vi "PID Servo Position.vi"() -> ()   [LabVIEW 2012]
doc: "<B>PID Servo Position</B> implements PID control of the Camera Servo Motor."
uses:
  <vilib>/Rock Robotics/SystemInterfaces/DIO/FPGA_DIOPWMChannel.ctl
  <vilib>/Rock Robotics/SystemInterfaces/Typedef/FPGA_TypedefDigitalModule.ctl
  <vilib>/addons/control/pid/pid.llb/PID (DBL).vi
  <vilib>/addons/control/pid/NI_PID_pid.lvlib
panel:
  in  "PID gains":T1={"proportional gain (Kc)"=1.0, "integral time (Ti, min)"=0.01, "derivative time (Td, min)"=0.0} {"derivative time (Td, min)" format="%.3f"; "integral time (Ti, min)" format="%.3f"; "proportional gain (Kc)" format="%.3f"}
  in  "Desired Angle":dbl format="%.2f"
  in  "PWM Channel":T2=enum."PWM 6"
  out "Current Angle":u16(knob) scale=0.0..170.0
  in  "stop":bool
  # "1. Select the PWM channel for the servo.\n2. Press the run button\n3. Adjust the PID Gains\n4. Set your Desired Angle\n5. The Current Angle is displayed in the dial\n6. Press STOP to end the program"
  # "Wiring Diagram for Digital Sidecar connected to an NI 9403"
  # "power jumper required for servo"
  # "The black wire should go into ground (-).\nThe red wire should go to power (PWR)\nThe white or yellow wire should go to signal (SIG)"
  # "PWR"
  # "SIG"
  # "(-)"
  # "+V"
  # "10"
  # "9"
  # "8"
  # "7"
  # "6"
  # "5"
  # "4"
  # "3"
  # "2"
  # "1"
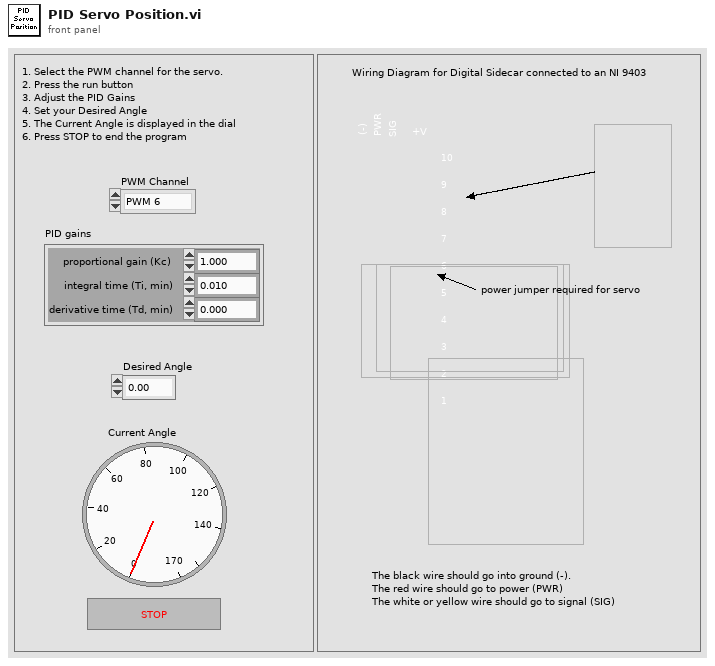
[diagram p1: front panel]
types:
  T1 = cluster{"proportional gain (Kc)":dbl, "integral time (Ti, min)":dbl, "derivative time (Td, min)":dbl}
  T2 = typedef "FPGA_DIOPWMChannel.ctl" = enum8{"PWM 1", "PWM 2", "PWM 3", "PWM 4", "PWM 5", "PWM 6", "PWM 7", "PWM 8", "PWM 9", "PWM 10", "Invalid"}
  T3 = typedef "FPGA_TypedefDigitalModule.ctl" = enum16{"Digital Module 1", "Digital Module 2"}
  T4 = typedef "WPI_ServoDeviceRef.ctl" = cluster{"DeviceStatus":errorcluster, "Digital Module":T3, "PWM Channel":T2, "DeadBand":T5}
  T5 = typedef "WPI_PWMDeadband.ctl" = cluster{"Name":string, "maxPositivePwm":i32, "minPositivePwm":i32, "centerPwm":i32, "maxNegativePwm":i32, "minNegativePwm":i32, "angularRange":u16}
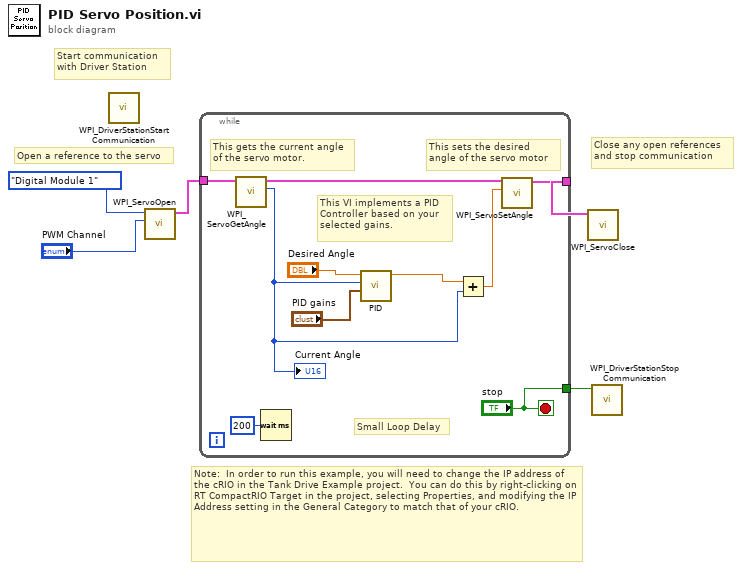
[diagram p0: block diagram]
diagram:
  # "Note:  In order to run this example, you will need to change the IP address of the cRIO in the Tank Drive Example project.  You can do this by right-clicking on RT CompactRIO Target in the project, selecting Properties, and modifying the IP Address setting in the General Category to match that of your cRIO."
  # "Close any open references\nand stop communication"
  # "Open a reference to the servo"
  # "Start communication\nwith Driver Station"
  n1 = call <vilib>:"WPI_DriverStationStart Communication.vi"() -> ()  [unwired: 12 in]
  n2 = call <vilib>:"WPI_ServoOpen.vi"("PWM Channel"="PWM Channel", "Digital Module (Module 1)"=FPGA_TypedefDigitalModule."Digital Module 1") -> ("ServoDeviceRef"=w3:T4)  [unwired: 8 in, 1 out]
  n3 = while {
    tunnel: w3 -> [w15]
    tunnel: [w8] -> w2
    tunnel: ["stop"] -> w1
    stop <- "stop" stop-if-true
    # "This VI implements a PID\nController based on your\nselected gains."
    # "This sets the desired\nangle of the servo motor"
    # "This gets the current angle\nof the servo motor."
    # "Small Loop Delay"
    n4 = call <vilib>:"WPI_ServoGetAngle.vi"("ServoDeviceRef"=w15) -> ("ServoDeviceRef"=w10:T4, "Angle"=w11:u16)  [unwired: 7 in, 1 out]
    "Current Angle" <- w11
    n5 = Wait (ms)(milliseconds to wait=u32 200) -> ()  [unwired: 1 out]
    n6 = call-poly <vilib>:"PID.vi"("PID gains"="PID gains", "process variable"=w11, "setpoint"="Desired Angle") -> ("output"=w12:dbl)  [unwired: 7 in, 1 out]
    n7 = Add(x=w12, y=w11) -> (x+y=w9:dbl)
    n8 = call <vilib>:"WPI_ServoSetAngle.vi"("Angle"=w9, "ServoDeviceRef"=w10) -> ("ServoDeviceRef"=w8:T4)  [unwired: 8 in, 1 out]
  }
  n9 = call <vilib>:"WPI_ServoClose.vi"("MotorControlDevRef"=w2) -> ()  [unwired: 10 in, 1 out]
  n10 = call <vilib>:"WPI_DriverStationStop Communication.vi"("StopCommunication"=w1) -> ()  [unwired: 10 in, 1 out]
